vi "Display Queue.vi"(7 "Action":T1=enum."Enqueue", 8 "error in (no error)":errorcluster, 9 "max queue size (-1, unlimited)":i32=1, 10 "time out":i32=100, 11 "input data":sgl[][](array[numeric])) -> (0 "error out":errorcluster, 1 "timed out?":bool, 2 "Empty?":bool, 3 "output data":sgl[][](array[numeric]), 5 "# elements in queue":i32)   [LabVIEW 2018]
uses:
  Controls/Queue Manager Actions.ctl
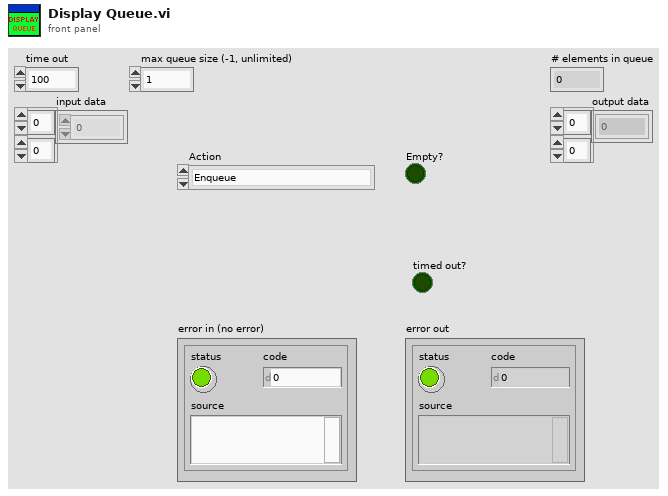
[diagram p1: front panel]
types:
  T1 = typedef "Queue Manager Actions.ctl" = enum16{"Init", "Enqueue", "Enqueue All", "Preview Queue", "Dequeue", "Get Status", "Flush Queue", "Flush All Queues", "Release All Queues", "Release Queue", "Enqueue at Opposite End"}
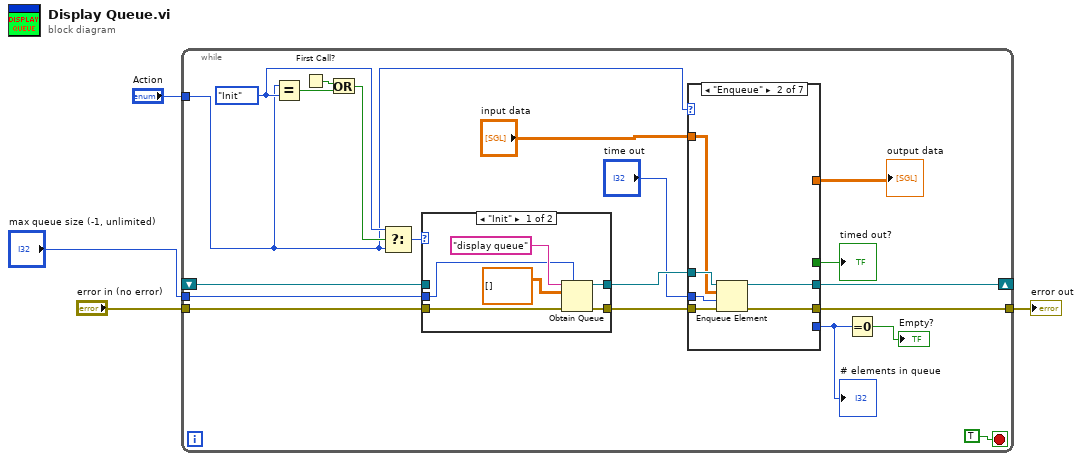
[diagram p0: block diagram]
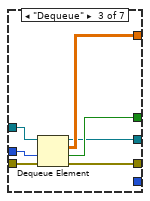
[diagram p3: hidden frame]
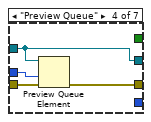
[diagram p4: hidden frame]
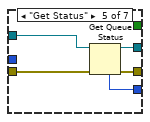
[diagram p5: hidden frame]
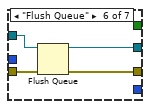
[diagram p6: hidden frame]
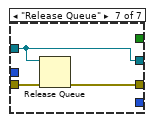
[diagram p7: hidden frame]
diagram:
  n1 = while {
    tunnel: "Action" -> [w12]
    tunnel: "error in (no error)" -> [w19]
    tunnel: [w18] -> w2
    shift-right: [w14] -> _
    shift-left: _ -> [w13]
    tunnel: "max queue size (-1, unlimited)" -> [w7]
    stop <- TRUE stop-if-true
    w21 = Queue_Manager_Actions."Init"
    n2 = Equal?(x=w12, y=w21) -> (x = y?=w23:bool)
    n3 = First Call?() -> (First Call?: T/F=w24:bool)
    n4 = Or(x=w24, y=w23) -> (x .or. y?=w22:bool)
    n5 = Select(t=w21, s=w22, f=w12) -> (s? t:f=w20:T1)
    n6 = case shown="\"Init\"" w20 {
      tunnel: [w61 w62] -> w16
      tunnel: w19 -> [w60 w63]
      tunnel: [w59 w63] -> w17
      tunnel: w13 -> [_ w62]
      tunnel: w7 -> [w56 _]
      frame "Init" {
        n7 = Obtain Queue(max queue size (-1, unlimited)=w56, name (unnamed)="display queue" ("queue name"), element data type=sgl[][] [], error in (no error)=w60) -> (queue out=w61:refnum<queue>, error out=w59:errorcluster)  [unwired: 1 in, 1 out]
      }
      frame "Enqueue", Default {
      }
    }
    n8 = case shown="\"Enqueue\"" w12 {
      tunnel: w16 -> [w25 w30 w37 w40 w46 w50 w53]
      tunnel: [w26 w27 w33 w42 w47 w51 w54] -> w18
      tunnel: w17 -> [w26 w32 w39 w43 w48 w52 w55]
      tunnel: [w25 w28 w34 w40 w45 w49 w53] -> w14
      tunnel: "time out" -> [_ w31 w38 w41 _ _ _]
      tunnel: [_ _ _ _ w44 _ _] -> w10
      tunnel: [_ _ w36 _ _ _ _] -> w9
      tunnel: "input data" -> [_ w29 _ _ _ _ _]
      tunnel: [_ _ w35 _ _ _ _] -> w5
      frame "Init", Default {
      }
      frame "Enqueue" {
        n9 = Enqueue Element(queue=w30, element=w29, timeout in ms (-1)=w31, error in (no error)=w32) -> (queue out=w28:refnum<queue>, error out=w27:errorcluster)  [unwired: 1 out]
      }
      frame "Dequeue" {
        n10 = Dequeue Element(queue=w37, timeout in ms (-1)=w38, error in (no error)=w39) -> (queue out=w34:refnum<queue>, element=w35:sgl[][], timed out?=w36:bool, error out=w33:errorcluster)
      }
      frame "Preview Queue" {
        n11 = Preview Queue Element(queue=w40, timeout in ms (-1)=w41, error in (no error)=w43) -> (error out=w42:errorcluster)  [unwired: 3 out]
      }
      frame "Get Status" {
        n12 = Get Queue Status(queue=w46, error in (no error)=w48) -> (queue out=w45:refnum<queue>, error out=w47:errorcluster, # elements in queue=w44:i32)  [unwired: 1 in, 5 out]
      }
      frame "Flush Queue" {
        n13 = Flush Queue(queue=w50, error in (no error)=w52) -> (queue out=w49:refnum<queue>, error out=w51:errorcluster)  [unwired: 1 out]
      }
      frame "Release Queue" {
        n14 = Release Queue(queue=w53, error in (no error)=w55) -> (error out=w54:errorcluster)  [unwired: 1 in, 2 out]
      }
    }
    "timed out?" <- w9
    "# elements in queue" <- w10
    "output data" <- w5
    n15 = Equal To 0?(x=w10) -> (x = 0?=→"Empty?":bool)
  }
  "error out" <- w2
